vi "SingleAxisMoveZIncremental.vi"(5 "Distance":dbl, 6 "stop":bool, 7 "Speed":dbl, 9 "\"FIX U\"":string, 11 "AxisName":string) -> (3 "Z Incremental Position":string)   [LabVIEW 2016]
uses:
  Examples/Motion/EnableSingle.vi
  Examples/Motion/MoveIncSingle.vi
  Examples/Motion/WaitSingle.vi
  Examples/Motion/DisableSingle.vi
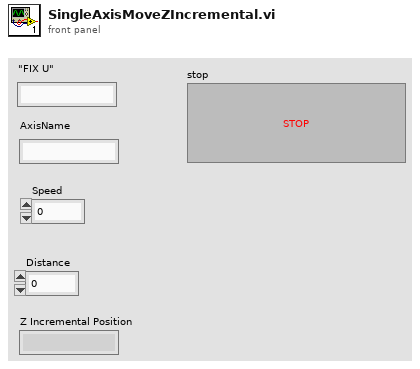
[diagram p1: front panel]
types:
  T1 = typedef "ControllerDiagPacket.ctl" = cluster{"Number of Diag Packets":i32, "Axes":T2[], "error":errorcluster}
  T2 = typedef "AxisDiagPacket.ctl" = cluster{"Axis Name":string, "Analog Input 0":dbl, "Analog Input 1":dbl, "Axis Fault (num)":i32, "Axis Fault (str)":string, "Axis Fault (bits)":cluster{"AmplifierFault":bool, "AmplifierTemperatureFault":bool, "CcwEndOfTravelLimitFault":bool, "CcwSoftwareLimitFault":bool, "CommunicationLostFault":bool, "CwEndOfTravelLimitFault":bool, "CwSoftwareLimitFault":bool, "EmergencyStopFault":bool, "EncoderFault":bool, "ExternalFault":bool, "FeedbackScalingFault":bool, "GantryMisalignFault ":bool, "HallSensorFault":bool, "InPositionTimeoutFault":bool, "MarkerSearchFault":bool, "MaxVelocityCommandFault":bool, "MissedInterruptFault":bool, "MotorTemperatureFault":bool, "None":bool, "OverCurrentFault":bool, "PositionErrorFault":bool, "PositionFeedbackFault":bool, "PowerSupplyFault":bool, "ProbeInputFault":bool, "SafeZoneFault":bool, "VelocityErrorFault":bool, "VelocityFeedbackFault":bool, "VoltageClampFault":bool}, "Axis Status (num)":i32, "Axis Status (str)":string, "Axis Status (bits)":cluster{"BacklashActive":bool, "CalibrationEnabled1D":bool, "CalibrationEnabled2D":bool, "CommandValid":bool, "DriveAbortPending":bool, "DrivePending":bool, "Enabling":bool, "GainMappingEnabled":bool, "GantryAligned":bool, "GantryRealigning":bool, "Homed":bool, "Homing":bool, "IFOVEnabled":bool, "JogGenerating":bool, "Jogging":bool, "JoystickControl":bool, "MasterSlaveControl":bool, "MotionBlocked":bool, "MotionClamped":bool, "MoveDone":bool, "None":bool, "NotVirtual":bool, "Profiling":bool, "Stability0":bool, "Stability1":bool, "TrajectoryFiltering":bool, "WaitDone":bool}, "Current Command":sgl, "Current Error":sgl, "Current Feedback":sgl, "Digital Inputs":i32, "Digital Outputs":i32, "Drive Status":i32, "Drive Status (str)":string, "Drive Status (bits)":cluster{"AccelerationPhase":bool, "AutofocusActive":bool, "BrakeOutput":bool, "CcwEndOfTravelLimitInput":bool, "CosineEncoderError":bool, "CurrentClamp":bool, "CwEndOfTravelLimitInput":bool, "DecelerationPhase":bool, "DualLoopActive":bool, "EmergencyStopInput":bool, "Enabled":bool, "EncoderClipping":bool, "GalvoCalibrationEnabled":bool, "GalvoPowerCorrection":bool, "HallAInput":bool, "HallBInput":bool, "HallCInput":bool, "HighResolutionMode":bool, "HomeLimitInput":bool, "InPosition":bool, "InPosition2":bool, "MarkerInput":bool, "MarkerLatch":bool, "MoveActive":bool, "NoMotorSupply":bool, "None":bool, "PowerLimiting":bool, "ProgrammingFlash":bool, "ProgrammingMXH":bool, "PSOHaltLatch":bool, "ServoControl":bool, "SineEncoderError":bool}, "Position Feedback Auxiliary":dbl, "Position Command":dbl, "Position Error":dbl, "Position Feedback":dbl, "Program Position Command":dbl, "Program Position Error":dbl, "Program Position Feedback":dbl, "Velocity Command":dbl, "Velocity Error":dbl, "Velocity Feedback":dbl}
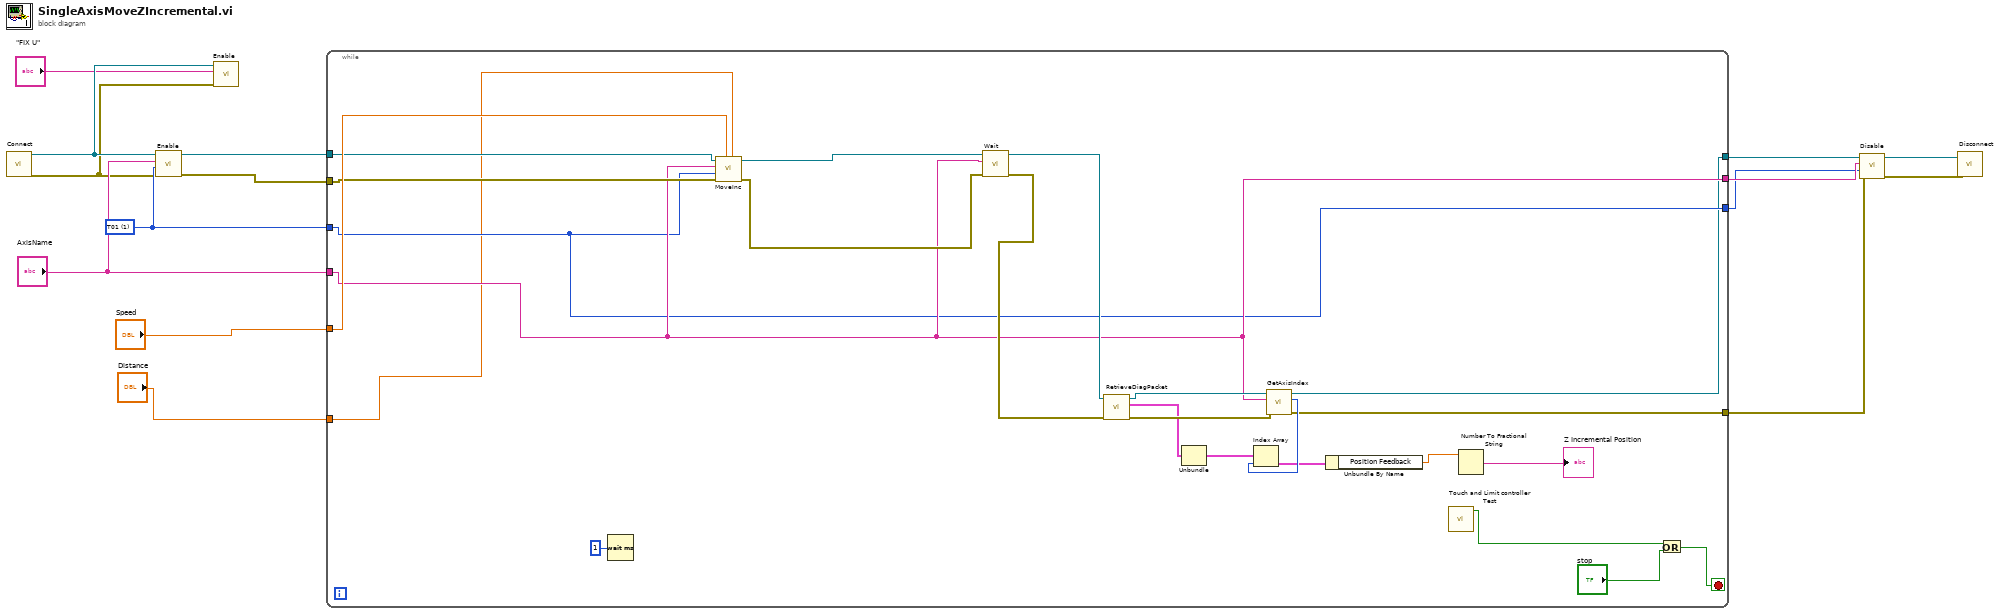
[diagram p0: block diagram]
diagram:
  w10 = 1 items=["TLibrary", "T01", "T02", "T03", "T04", "T05", "T06", "T07", "T08", "T09", "T10", "T11", "T12", "T13", "T14", "T15", "T16", "T17", "T18", "T19", "T20", "T21", "T22", "T23", "T24", "T25", "T26", "T27", "T28", "T29", "T30", "T31"] ("taskId")
  n1 = call "Connect.vi"() -> ("error out"=w2:errorcluster, "controller"=w3:refnum<k24>)  [unwired: 10 in]
  n2 = call-poly "Enable.vi"("error in (no error)"=w2, "taskId"=w10, "axis name"="AxisName", "controller in"=w3) -> ("error out"=w11:errorcluster, "controller out"=w13:refnum<k24>)  [unwired: 6 in]
  n3 = call-poly "Enable.vi"("error in (no error)"=w2, "axis name"="\"FIX U\"", "controller in"=w3) -> ()  [unwired: 7 in, 2 out]
  n4 = while {
    tunnel: w13 -> [w25]
    tunnel: "AxisName" -> [w23]
    tunnel: "Speed" -> [w27]
    tunnel: "Distance" -> [w19]
    tunnel: w10 -> [w22]
    tunnel: w11 -> [w26]
    tunnel: [w20] -> w9
    tunnel: [w23] -> w7
    tunnel: [w22] -> w6
    tunnel: [w21] -> w5
    stop <- w16 stop-if-true
    n5 = Wait (ms)(milliseconds to wait=u32 1) -> ()  [unwired: 1 out]
    n6 = call-poly "MoveInc.vi"("distance"=w19, "speed"=w27, "error in (no error)"=w26, "taskId"=w22, "axis name"=w23, "controller in"=w25) -> ("error out"=w39:errorcluster, "controller out"=w38:refnum<k24>)  [unwired: 4 in]
    n7 = call-poly "Wait.vi"("error in (no error)"=w39, "axis name"=w23, "controller in"=w38) -> ("error out"=w37:errorcluster, "controller out"=w24:refnum<k24>)  [unwired: 6 in, 1 out]
    n8 = call "RetrieveDiagPacket.vi"("error in (no error)"=w37, "Controller In"=w24) -> ("error out"=w36:errorcluster, "ControllerDiagPacket"=w34:T1, "Controller Out"=w35:refnum<k24>)  [unwired: 7 in]
    n9 = Unbundle(w34) -> ("Axes"=w33:T2[])  [unwired: 2 out]
    n10 = call "GetAxisIndex.vi"("error in (no error)"=w36, "axis name"=w23, "controller in"=w35) -> ("error out"=w21:errorcluster, "axis index"=w32:i32, "controller out"=w20:refnum<k24>)  [unwired: 6 in]
    n11 = Index Array(array=w33, index=w32) -> (element=w31:T2)
    n12 = Unbundle By Name(w31) -> ("Position Feedback"=w30:dbl)
    n13 = call "Touch and Limit controller Test.vi"() -> ("Touching"=w18:bool)  [unwired: 4 in, 1 out]
    n14 = Number To Fractional String(number=w30) -> (F-format string=→"Z Incremental Position":string)  [unwired: 3 in]
    n15 = Or(x=w18, y="stop") -> (x .or. y?=w16:bool)
  }
  n16 = call-poly "Disable.vi"("error in (no error)"=w5, "taskId"=w6, "axis name"=w7, "controller in"=w9) -> ("error out"=w4:errorcluster, "controller out"=w8:refnum<k24>)  [unwired: 6 in]
  n17 = call "Disconnect.vi"("error in (no error)"=w4, "controller"=w8) -> ()  [unwired: 9 in, 1 out]
